vi "FG FPGA Reference.vi"(2 "FG Action":T1, 3 "FPGA VI Reference in":T2) -> (1 "FPGA VI Reference out":T2)   [LabVIEW 2009]
uses:
  TypeDefs/Sensor Typedefs/FPGA Main ref.ctl
  Actions for FG's.ctl
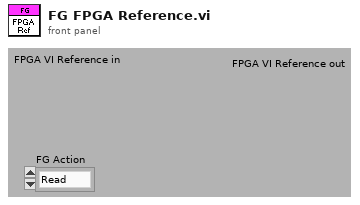
[diagram p1: front panel]
types:
  T1 = typedef "Actions for FG's.ctl" = enum16{"Read", "Write"}
  T2 = typedef "FPGA Main ref.ctl" = refnum<k20>
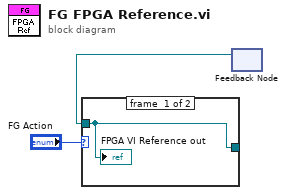
[diagram p0: block diagram]
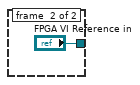
[diagram p2: hidden frame]
diagram:
  n1 = feedback #1() -> (w1:T2)  [unwired: 1 in]
  n2 = case shown="\"Read\", Default" "FG Action" {
    tunnel: w1 -> [w4 _]
    tunnel: [w4 "FPGA VI Reference in"] -> w2
    frame #0 {
      "FPGA VI Reference out" <- w4
    }
    frame #1 {
    }
  }
